vi "flower.vi"() -> ()   [LabVIEW 2021]
uses:
  <vilib>/Math Plots/3D Math Plots/3D Surface/3D Surface XCtrl/3D Surface.xctl
  <vilib>/Analysis/1siggen.llb/Ramp Pattern by Samples.vi
  <vilib>/gmath/interp.llb/Create Mesh Grid (2D) (x,y arrays).vi
  <vilib>/Math Plots/3D Math Plots/3D Surface/3D Surface Datatype/Public/Plot Helper (Matrix).vi
  <vilib>/Analysis/NI_AALBase.lvlib
  <vilib>/gmath/NI_Gmath.lvlib
  <vilib>/Math Plots/3D Math Plots/3D Surface/3D Surface Datatype/3D Surface Datatype.lvclass
panel:
  out "3D Surface":refnum<class "3D Plot Datatype.lvclass">[](xcontrol)
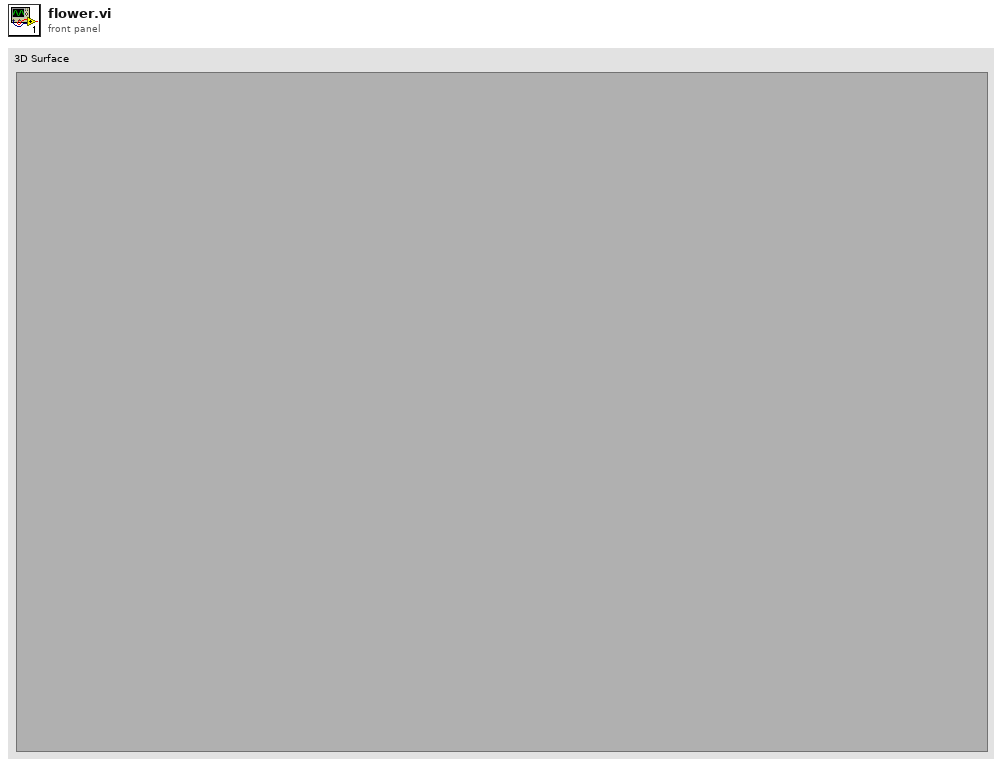
[diagram p1: front panel]
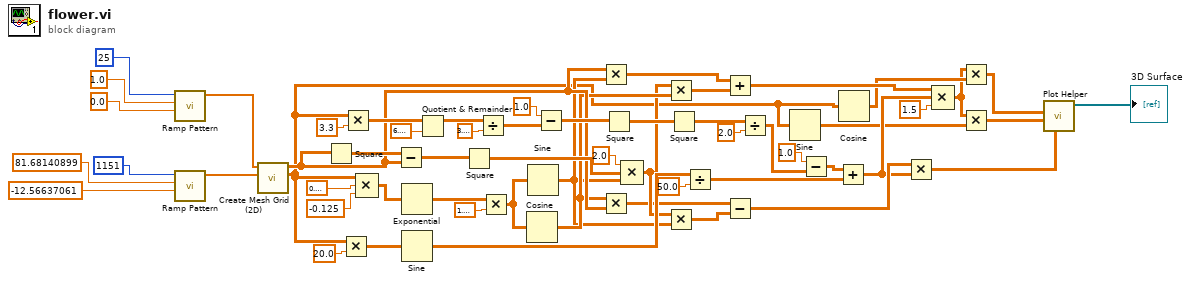
[diagram p0: block diagram]
diagram:
  n1 = call-poly <vilib>:"Ramp Pattern.vi"("start"=0.0, "end"=1.0, "samples"=25) -> ("Ramp Pattern"=w51:dbl[])  [unwired: 7 in, 1 out]
  n2 = call-poly <vilib>:"Ramp Pattern.vi"("start"=-12.56637061, "end"=81.68140899, "samples"=1151) -> ("Ramp Pattern"=w50:dbl[])  [unwired: 7 in, 1 out]
  n3 = call-poly <vilib>:"Create Mesh Grid (2D).vi"("y domain"=w50, "x domain"=w51) -> ("Y"=w6:dbl[][], "X"=w18:dbl[][])  [unwired: 7 in, 1 out]
  n4 = Square(x=w18) -> (x^2=w25:dbl[][])
  n5 = Multiply(x=w6, y=20.0 ("value")) -> (x*y=w43:dbl[][])
  n6 = Multiply(x=w6, y=3.3 ("value")) -> (x*y=w38:dbl[][])
  n7 = Compound Arithmetic op=MULTIPLY(w6, 0.3183098861837907, -0.125 ("value")) -> (w47:dbl[][])
  n8 = Subtract(x=w25, y=w18) -> (x-y=w24:dbl[][])
  n9 = Exponential(1:w47) -> (0:w46:dbl[][])
  n10 = Sine(x=w43) -> (sin(x)=w42:dbl[][])
  n11 = Quotient & Remainder(x=w38, y=6.283185307179586) -> (x-y*floor(x/y)=w37:dbl[][])  [unwired: 1 out]
  n12 = Square(x=w24) -> (x^2=w23:dbl[][])
  n13 = Divide(x=w37, y=3.141592653589793) -> (x/y=w27:dbl[][])
  n14 = Multiply(x=w46, y=1.5707963267948966) -> (x*y=w21:dbl[][])
  n15 = Cosine(x=w21) -> (cos(x)=w17:dbl[][])
  n16 = Sine(x=w21) -> (sin(x)=w15:dbl[][])
  n17 = Subtract(x=1.0, y=w27) -> (x-y=w26:dbl[][])
  n18 = Multiply(x=w18, y=w15) -> (x*y=w20:dbl[][])
  n19 = Multiply(x=w17, y=w18) -> (x*y=w14:dbl[][])
  n20 = Square(x=w26) -> (x^2=w35:dbl[][])
  n21 = Compound Arithmetic op=MULTIPLY(2.0 ("value"), w23, w15) -> (w16:dbl[][])
  n22 = Multiply(x=w16, y=w17) -> (x*y=w19:dbl[][])
  n23 = Multiply(x=w16, y=w15) -> (x*y=w13:dbl[][])
  n24 = Square(x=w35) -> (x^2=w34:dbl[][])
  n25 = Divide(x=w42, y=50.0 ("value")) -> (x/y=w29:dbl[][])
  n26 = Add(x=w20, y=w19) -> (x+y=w12:dbl[][])
  n27 = Subtract(x=w14, y=w13) -> (x-y=w10:dbl[][])
  n28 = Divide(x=w34, y=2.0 ("value")) -> (x/y=w31:dbl[][])
  n29 = Sine(x=w6) -> (sin(x)=w4:dbl[][])
  n30 = Subtract(x=1.0, y=w31) -> (x-y=w30:dbl[][])
  n31 = Add(x=w30, y=w29) -> (x+y=w9:dbl[][])
  n32 = Cosine(x=w6) -> (cos(x)=w8:dbl[][])
  n33 = Multiply(x=w10, y=w9) -> (x*y=w2:dbl[][])
  n34 = Compound Arithmetic op=MULTIPLY(w12, w9, 1.5 ("x")) -> (w5:dbl[][])
  n35 = Multiply(x=w5, y=w8) -> (x*y=w7:dbl[][])
  n36 = Multiply(x=w5, y=w4) -> (x*y=w3:dbl[][])
  n37 = call-poly <vilib>:"Plot Helper.vi"("z matrix"=w2, "y matrix"=w3, "x matrix"=w7) -> ("3D Plot lvclass Array out"=→"3D Surface":refnum<class "3D Plot Datatype.lvclass">[])  [unwired: 3 in, 5 out]
